vi "Pre Launch Init.vi"(11 "ObservingViewModel In":refnum<class "ObservingViewModel.lvclass">) -> (0 "error out":errorcluster, 3 "ObservingViewModel Out":refnum<class "ObservingViewModel.lvclass">)   [LabVIEW 2015, in "ObservingViewModel.lvclass"]
doc: "(<B>Filename</B>: Actor Framework.lvlib:Actor.lvclass:Pre Launch Init.vi)\n\nDefines behavior that occurs after the Launch Nested Actor method is invoked but before the actor's Actor Core method begins running.\n\nBy default, this method does nothing. A descendant class may override it to define behavior."
uses:
  ObservingViewModel.lvclass
  Framework/IViewModel/IViewModel/IViewModel.lvclass
  Framework/IObserver/IObserver/IObserver.lvclass
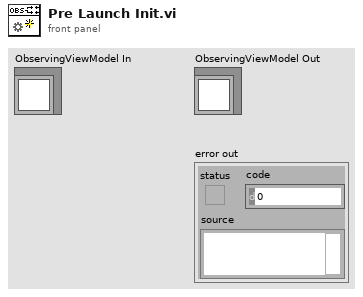
[diagram p1: front panel]
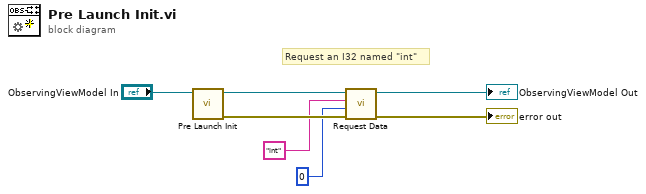
[diagram p0: block diagram]
diagram:
  # "Request an I32 named \"int\""
  n1 = call-parent "Pre Launch Init.vi"("IViewModel In"="ObservingViewModel In") -> ("error out"=w4:errorcluster, "IViewModel Out"=w7:refnum<class "ObservingViewModel.lvclass">)  [unwired: 9 in]
  n2 = call "Request Data.vi"("error in (no error)"=w4, "Data Type"=0, "Datum Name"="int", "IObserver in"=w7) -> ("error out"=→"error out":errorcluster, "IObserver out"=→"ObservingViewModel Out":refnum<class "ObservingViewModel.lvclass">)  [unwired: 5 in, 1 out]
